vi "ReadWriteConfigTool.vi"() -> ()   [LabVIEW 2012]
uses:
  Controls/Config.ctl
  <vilib>/Utility/error.llb/DialogType.ctl
  <vilib>/Utility/config.llb/Read Key (I32).vi
  <vilib>/Utility/config.llb/Read Key (Double).vi
  <vilib>/Utility/config.llb/Write Key (I32).vi
  <vilib>/Utility/config.llb/Write Key (Double).vi
  <vilib>/Utility/config.llb/NI_LVConfig.lvlib
panel:
  in  "error IO":errorcluster
  in  "Configuration":T1={"IntTime"=100, "Samples"=3, "PowerMin"=400.0, "KneeMin"=-20.0, "KneeMax"=20.0, "Background Wl"=275.0, "Settle Delay,ms"=275, "StationId"=1.0} {"Background Wl" min=220.0 max=320.0; "IntTime" min=1 max=100000; "PowerMin" min=0.0 max=10000.0; "KneeMin" min=-40.0 max=0.0; "KneeMax" min=0.0 max=40.0; "Samples" min=1 max=10}
  in  "Action":enum16{"Read", "Write"}(ring)
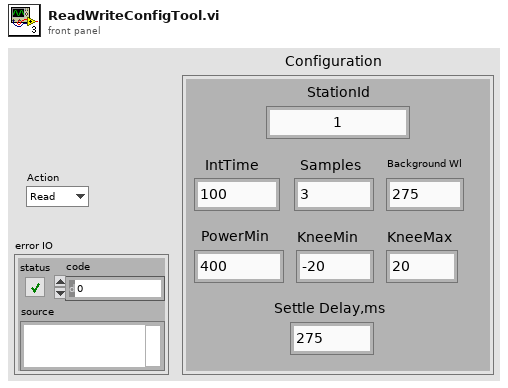
[diagram p1: front panel]
types:
  T1 = typedef "Config.ctl" = cluster{"IntTime":i32, "Samples":i32, "PowerMin":dbl, "KneeMin":dbl, "KneeMax":dbl, "Background Wl":dbl, "Settle Delay,ms":u32, "StationId":sgl}
  T2 = typedef "DialogType.ctl" = u16
  T3 = typedef "NI_LVConfig.lvlib/Config Data RefNum.ctl" = refnum<k1>
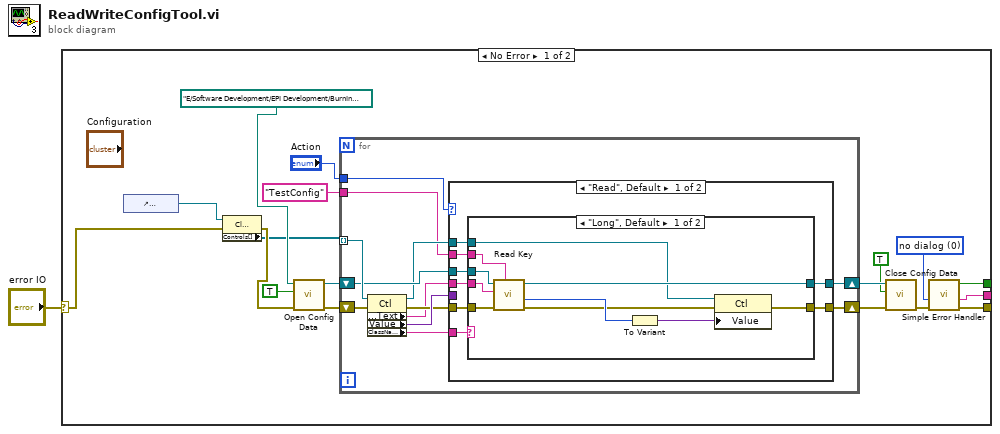
[diagram p0: block diagram]
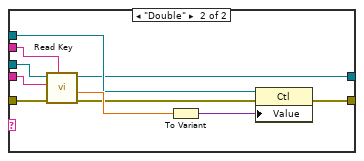
[diagram p2: hidden frame]
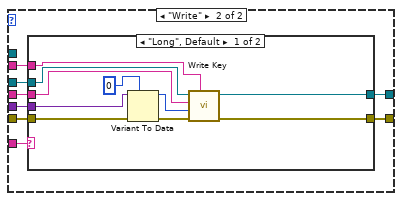
[diagram p3: hidden frame]
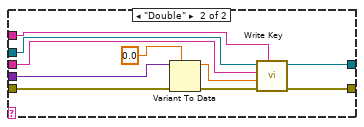
[diagram p4: hidden frame]
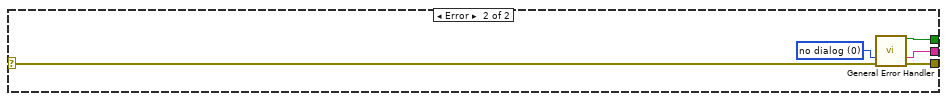
[diagram p5: hidden frame]
diagram:
  n1 = case shown="No Error" "error IO" {
    selector: "error IO" -> [w4 w92]
    tunnel: [w8 w90] -> _
    tunnel: [w10 w88] -> _
    tunnel: [w9 w89] -> _
    frame No Error {
      w11 = T2 0 items=["no dialog", "OK message", "continue or stop message", "OK message + warnings", "continue/stop + warnings"] ("type of dialog (OK msg:1)")
      n2 = control-ref of="Configuration"() -> (w5:refnum<vi>)
      n3 = property class="Clust (strict)"(reference=w5, error in=w4) -> (error out=w3:errorcluster, "Controls[]"=w2:refnum<vi>[])  [unwired: 1 out]
      n4 = call <vilib>:"Open Config Data.vi"("error in (no error)"=w3, "create file if necessary (T)"=TRUE, "configuration file path"=path "E:/Software Development/EPI Development/BurnIn Testing/Resources/TestConfiguration.cfg") -> ("error out"=w18:errorcluster, "refnum"=w19:T3)  [unwired: 6 in, 1 out]
      n5 = for {
        tunnel: w2 -> [w31] mode=indexing
        shift-right: [w26] -> w15
        shift-left: w18 -> [w27]
        shift-right: [w25] -> w17
        shift-left: w19 -> [w28]
        tunnel: "Action" -> [w24]
        tunnel: "TestConfig" ("section") -> [w22]
        n6 = property class="Ctl"(reference=w31, error in=w27) -> (reference out=w23:refnum<vi>, error out=w29:errorcluster, "Label.Text"=w20:string, "Value"=w30:variant, "ClassName"=w21:string)
        n7 = case shown="\"Read\", Default" w24 {
          tunnel: w30 -> [_ w67]
          tunnel: w29 -> [w38 w66]
          tunnel: w28 -> [w39 w65]
          tunnel: [w36 w64] -> w26
          tunnel: [w35 w63] -> w25
          tunnel: w23 -> [w37 _]
          tunnel: w22 -> [w33 w62]
          tunnel: w21 -> [w34 w61]
          tunnel: w20 -> [w32 w60]
          frame "Read", Default {
            n8 = case shown="\"Long\", Default" w34 {
              tunnel: [w42 w52] -> w36
              tunnel: [w47 w53] -> w35
              tunnel: w39 -> [w49 w56]
              tunnel: w38 -> [w48 w54]
              tunnel: w37 -> [w44 w55]
              tunnel: w33 -> [w41 w51]
              tunnel: w32 -> [w40 w50]
              frame "Long", Default {
                n9 = call-poly <vilib>:"Read Key.vi"("section"=w41, "error in (no error)"=w48, "key"=w40, "refnum"=w49) -> ("error out"=w43:errorcluster, "value"=w45:i32, "refnum out"=w47:T3)  [unwired: 1 in, 4 out]
                n10 = To Variant(anything=w45) -> (Variant=w46:variant)
                n11 = property class="Ctl"(reference=w44, error in=w43, "Value"=w46) -> (error out=w42:errorcluster)  [unwired: 1 out]
              }
              frame "Double" {
                n12 = call-poly <vilib>:"Read Key.vi"("section"=w51, "error in (no error)"=w54, "key"=w50, "refnum"=w56) -> ("error out"=w57:errorcluster, "value"=w58:dbl, "refnum out"=w53:T3)  [unwired: 1 in, 4 out]
                n13 = To Variant(anything=w58) -> (Variant=w59:variant)
                n14 = property class="Ctl"(reference=w55, error in=w57, "Value"=w59) -> (error out=w52:errorcluster)  [unwired: 1 out]
              }
            }
          }
          frame "Write" {
            n15 = case shown="\"Long\", Default" w61 {
              tunnel: w67 -> [w77 w86]
              tunnel: w66 -> [w75 w85]
              tunnel: [w72 w81] -> w64
              tunnel: w65 -> [w71 w82]
              tunnel: [w70 w80] -> w63
              tunnel: w62 -> [w69 w79]
              tunnel: w60 -> [w68 w78]
              frame "Long", Default {
                n16 = Variant To Data(error in=w75, type=0, Variant=w77) -> (data=w74:i32, error out=w73:errorcluster)
                n17 = call-poly <vilib>:"Write Key.vi"("section"=w69, "error in (no error)"=w73, "value"=w74, "key"=w68, "refnum"=w71) -> ("error out"=w72:errorcluster, "refnum out"=w70:T3)  [unwired: 4 in, 1 out]
              }
              frame "Double" {
                n18 = Variant To Data(error in=w85, type=0.0, Variant=w86) -> (data=w84:dbl, error out=w83:errorcluster)
                n19 = call-poly <vilib>:"Write Key.vi"("section"=w79, "error in (no error)"=w83, "value"=w84, "key"=w78, "refnum"=w82) -> ("error out"=w81:errorcluster, "refnum out"=w80:T3)  [unwired: 4 in, 1 out]
              }
            }
          }
        }
      }
      n20 = call <vilib>:"Close Config Data.vi"("error in (no error)"=w15, "write file if changed (T)"=TRUE, "refnum"=w17) -> ("error out"=w12:errorcluster)  [unwired: 8 out]
      n21 = call <vilib>:"Simple Error Handler.vi"("type of dialog (OK msg:1)"=w11, "error in (no error)"=w12) -> ("error?"=w10:bool, "source out"=w9:string, "error out"=w8:errorcluster)  [unwired: 3 in, 2 out]
    }
    frame Error {
      w91 = T2 0 items=["no dialog", "OK message", "continue or stop message", "OK message + warnings", "continue/stop + warnings"] ("type of dialog (OK msg:1)")
      n22 = call <vilib>:"General Error Handler.vi"("type of dialog (OK msg:1)"=w91, "error in (no error)"=w92) -> ("error?"=w88:bool, "message"=w89:string, "error out"=w90:errorcluster)  [unwired: 9 in, 2 out]
    }
  }
